vi "xiUtils - ExeVersion.vi"() -> (7 "File Version Info":string)   [LabVIEW 2015]
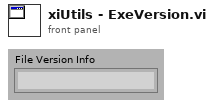
[diagram p1: front panel]
types:
  T1 = enum32{"invalid app kind", "Development System", "Run Time System", "Student Edition", "Embedded LabVIEW", "Evaluation", "Custom"}
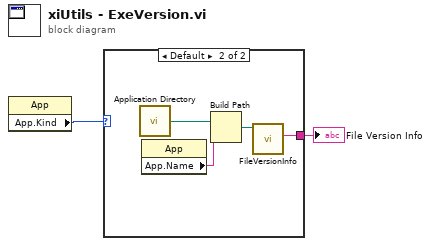
[diagram p0: block diagram]
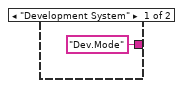
[diagram p2: hidden frame]
diagram:
  n1 = property class="App"() -> ("App.Kind"=w1:T1)  [unwired: 2 in, 2 out]
  n2 = case shown="Default" w1 {
    tunnel: ["Dev.Mode" ("File Version Info") w4] -> w2
    frame "Development System" {
    }
    frame Default {
      n3 = call <vilib>:"Application Directory.vi"() -> ("Application Directory"=w7:path)
      n4 = property class="App"() -> ("App.Name"=w6:string)  [unwired: 2 in, 2 out]
      n5 = Build Path(base path=w7, name or relative path=w6) -> (appended path=w5:path)
      n6 = call <vilib>:"FileVersionInfo.vi"("Application Path in"=w5) -> ("File Version Info"=w4:string)  [unwired: 7 in, 3 out]
    }
  }
  "File Version Info" <- w2
